vi "Lifschitz-Kosevich fit.vi"(9 "Temp":dbl[](array[numeric]), 10 "FFT":dbl[](array[numeric]), 11 "initial parameters":dbl[](array[numeric])) -> (2 "best fit parameters":dbl[](array[numeric]), 3 "best nonlinear fit":dbl[](array[numeric]))   [LabVIEW 2019]
uses:
  <vilib>/gmath/NumericalOptimization/Nonlinear Curve Fit LM.vi
  <vilib>/gmath/NI_Gmath.lvlib
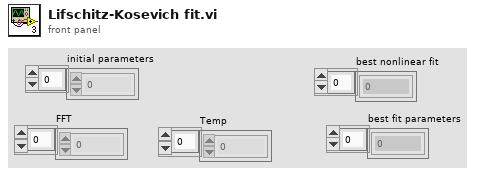
[diagram p1: front panel]
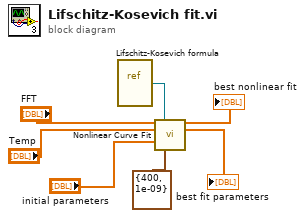
[diagram p0: block diagram]
diagram:
  n1 = vi-ref "Lifschitz-Kosevich formula.vi"() -> (w5:refnum<vi>)
  n2 = call-poly <vilib>:"Nonlinear Curve Fit.vi"("Y"="FFT", "f(x,a)"=w5, "X"="Temp", "initial parameters"="initial parameters", "termination"=cluster{"max iteration":i32, "tolerance":dbl} {"max iteration"=400, "tolerance"=1e-09}) -> ("best nonlinear fit"=→"best nonlinear fit":dbl[], "best fit parameters"=→"best fit parameters":dbl[])  [unwired: 5 in, 4 out]
